vi "controllerMain.vi"(8 "error in (no error)":errorcluster, 10 "UserEvents in":refnum<class "UserEvents.lvclass">, 11 "Controller in":refnum<class "Controller.lvclass">) -> (0 "error out":errorcluster, 3 "Controller out":refnum<class "Controller.lvclass">)   [LabVIEW 2013, in "Controller.lvclass"]
uses:
  Controller.lvclass
  UserEvents/UserEvents.lvclass
  StateFactory/StateFactory.lvclass
  Typedefs/StateSelector.ctl
  Model/Model/Model.lvclass
  Context/Context.lvclass
  CommandFactory/CommandFactory.lvclass
  <userlib>/Common/SerialProtocols/SerialProtocolFactory/SerialProtocolFactory/SerialProtocolFactory.lvclass
  <userlib>/Common/SerialProtocols/SerialCommunicator/SerialCommunicator.lvclass
  Model/ApplicationElements/ApplicationElements.ctl
  Model/ApplicationElements/Log/TestDataLog/TestDataLog.lvclass
  Model/ILCTC/ILCTC.lvclass
  Model/ILCSim1TC/ILCSim1TC.lvclass
  <userlib>/Common/SerialProtocols/SerialCommunicator/SerialCommunicator.lvclass/SerialCommunicator.ctl
  <userlib>/Common/ILC/ILC/ILC.lvclass/ILC.ctl
  Model/Model/Model.lvclass/Model.ctl
  UserEvents/UserEvents.lvclass/UserEvents.ctl
  Context/Context.lvclass/Context.ctl
  Command/Command.lvclass
  Typedefs/ILCBTTypedefs.lvlib
  <userlib>/Common/ILC/ILC/ILC.lvclass
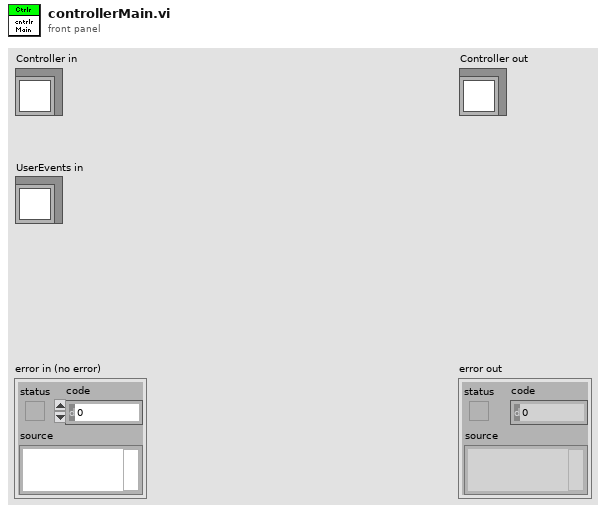
[diagram p1: front panel]
types:
  T1 = typedef "ApplicationElements.ctl" = cluster{"testDataLog":refnum<class "TestDataLog.lvclass">}
  T2 = typedef "ILCBTTypedefs.lvlib/StateSelector.ctl" = enum16{"EnabledState", "FaultState", "OffState", "StandbyState"}
  T3 = typedef "ILCBTTypedefs.lvlib/SubDataEvents.ctl" = cluster{"Command":refnum<user-event>}
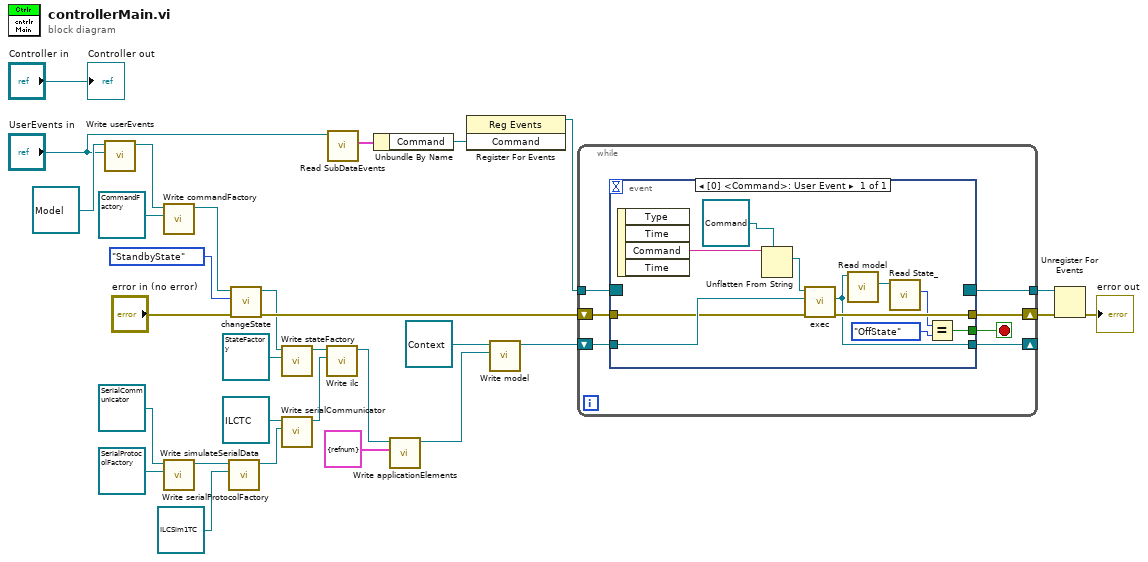
[diagram p0: block diagram]
diagram:
  n1 = call "Write userEvents.vi"("userEvents"="UserEvents in", "Model in"=refnum<class "Model.lvclass"> refnum) -> ("Model out"=w8:refnum<class "Model.lvclass">)  [unwired: 9 in]
  n2 = call "Write commandFactory.vi"("commandFactory"=refnum<class "CommandFactory.lvclass"> refnum ("CommandFactory.lvclass"), "Model in"=w8) -> ("Model out"=w6:refnum<class "Model.lvclass">)  [unwired: 9 in]
  n3 = call <userlib>:"Write serialProtocolFactory.vi"("serialProtocolFactory"=refnum<class "SerialProtocolFactory.lvclass"> refnum ("SerialCommFactory.lvclass"), "SerialCommunicator in"=refnum<class "SerialCommunicator.lvclass"> refnum ("SerialProtocols.lvlib:SerialCommunicator.lvclass")) -> ("SerialCommunicator out"=w14:refnum<class "SerialCommunicator.lvclass">)  [unwired: 9 in]
  n4 = call <userlib>:"Write simulateSerialData.vi"("simulateSerialData"=refnum<class "ILCSim1TC.lvclass"> refnum ("ILCSim1TC.lvclass"), "SerialCommunicator in"=w14) -> ("SerialCommunicator out"=w13:refnum<class "SerialCommunicator.lvclass">)  [unwired: 9 in]
  n5 = call "changeState.vi"("error in (no error)"="error in (no error)", "State:"=StateSelector."StandbyState", "Model in"=w6) -> ("error out"=w21:errorcluster, "Model out"=w4:refnum<class "Model.lvclass">)  [unwired: 7 in]
  n6 = call "Write stateFactory.vi"("stateFactory"=refnum<class "StateFactory.lvclass"> refnum ("StateFactory.lvclass"), "Model in"=w4) -> ("Model out"=w15:refnum<class "Model.lvclass">)  [unwired: 9 in]
  n7 = call <userlib>:"Write serialCommunicator.vi"("serialCommunicator"=w13, "ILC in"=refnum<class "ILCTC.lvclass"> refnum ("ILC_TC.lvclass")) -> ("ILC out"=w16:refnum<class "ILCTC.lvclass">)  [unwired: 9 in]
  n8 = call "Write ilc.vi"("ilc"=w16, "Model in"=w15) -> ("Model out"=w12:refnum<class "Model.lvclass">)  [unwired: 9 in]
  n9 = call "Read SubDataEvents.vi"("UserEvents in"="UserEvents in") -> ("SubDataEvents"=w25:T3)  [unwired: 9 in, 1 out]
  n10 = Unbundle By Name(w25) -> ("Command"=w19:refnum<user-event>)
  n11 = call "Write applicationElements.vi"("applicationElements"=T1 {"testDataLog"=refnum}, "Model in"=w12) -> ("Model out"=w11:refnum<class "Model.lvclass">)  [unwired: 9 in]
  n12 = register-events(w19) -> (reference out=w24:refnum<event-registration>)  [unwired: 2 in, 1 out]
  n13 = call "Write model.vi"("Model.lvclass"=w11, "Context in"=refnum<class "Context.lvclass"> refnum ("Context.lvclass")) -> ("Context out"=w27:refnum<class "Context.lvclass">)  [unwired: 9 in]
  n14 = while {
    shift-right: [w36] -> w22
    shift-left: w21 -> [w33]
    shift-right: [w35] -> _
    shift-left: w27 -> [w37]
    tunnel: w24 -> [w32]
    tunnel: [w31] -> w23
    stop <- w34 stop-if-true
    n15 = event shown="[0] <Command>: User Event" {
      selector: w32 -> [_]
      dyn-events: [_] -> w31
      timeout: _ -> [_]
      tunnel: w37 -> [w46]
      tunnel: [w43] -> w36
      tunnel: [w42] -> w35
      tunnel: [w41] -> w34
      tunnel: w33 -> [w39]
      event User Event {
        n16 = event-data() -> ("Command"=w38:string)  [unwired: 1 in, 3 out]
        n17 = Unflatten From String(type=refnum<class "Command.lvclass"> refnum ("Command.lvclass"), binary string=w38) -> (value=w47:refnum<class "Command.lvclass">)  [unwired: 3 in, 2 out]
        n18 = call-dynamic "exec.vi"("error in (no error)"=w39, "context"=w46, "Command in"=w47) -> ("error out"=w43:errorcluster, "context 2"=w42:refnum<class "Context.lvclass">)  [unwired: 6 in, 1 out]
        n19 = call "Read model.vi"("Context in"=w42) -> ("Model.lvclass"=w45:refnum<class "Model.lvclass">)  [unwired: 9 in, 1 out]
        n20 = call "Read State_.vi"("Model in"=w45) -> ("state:"=w40:T2)  [unwired: 9 in, 1 out]
        n21 = Equal?(x=w40, y=StateSelector."OffState") -> (x = y?=w41:bool)
      }
    }
  }
  n22 = Unregister For Events(event registration refnum=w23, error in=w22) -> (error out=→"error out":errorcluster)
  "Controller out" <- "Controller in"
